vi "Get AI Signals Properties.vi"(8 "error in (no error)":errorcluster, 11 "Item Ref in":T2 format="%.0x") -> (0 "error out":errorcluster, 1 "AI Signal properties Array":T1[](array[typedef]) {"Input Configuration" items=["RSE"=10083, "NRSE"=10078, "Differential"=10106]}, 3 "AI Signal Refs":T2[](array[typedef]) format="%.0x")   [LabVIEW 2021, in "DAQ Analog InOut System Explorer.lvlib"]
uses:
  DAQ Analog InOut System Explorer.lvlib
  <vilib>/NI VeriStand/Custom Device API/Custom Device Item Ref.ctl
  Types/Input Channel Parameters.ctl
  <vilib>/NI VeriStand/Custom Device API/Custom Device API.lvlib
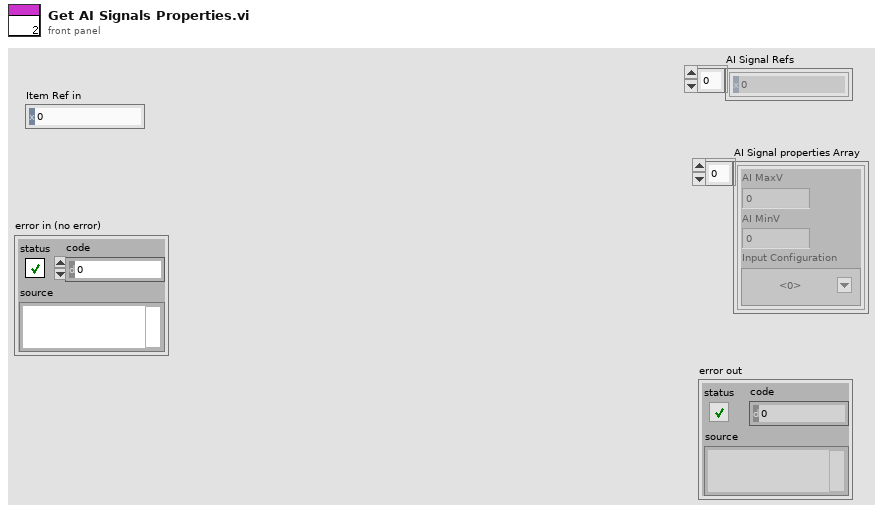
[diagram p1: front panel]
types:
  T1 = typedef "DAQ Analog InOut System Explorer.lvlib/Input Channel Parameters.ctl" = cluster{"AI MaxV":dbl, "AI MinV":dbl, "Input Configuration":u16}
  T2 = typedef "Custom Device API.lvlib/Custom Device Item Ref.ctl" = u64
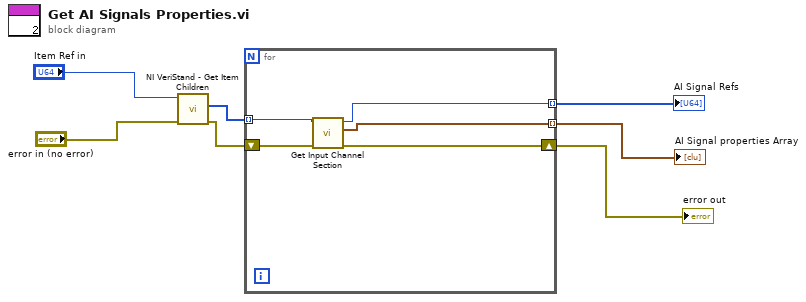
[diagram p0: block diagram]
diagram:
  n1 = call <vilib>:"NI VeriStand - Get Item Children.vi"("error in (no error)"="error in (no error)", "Item Ref in"="Item Ref in") -> ("error out"=w4:errorcluster, "Child Refs"=w5:T2[])  [unwired: 6 in, 2 out]
  n2 = for {
    tunnel: w5 -> [w12] mode=indexing
    shift-right: [w10] -> w2
    shift-left: w4 -> [w11]
    tunnel: [w9] -> w1 mode=indexing
    tunnel: [w8] -> w3 mode=indexing
    n3 = call "Get Input Channel Section.vi"("error in (no error)"=w11, "Ref in"=w12) -> ("error out"=w10:errorcluster, "Input Channel Parameters"=w9:T1, "Ref out"=w8:T2)  [unwired: 7 in]
  }
  "AI Signal Refs" <- w3
  "error out" <- w2
  "AI Signal properties Array" <- w1
